vi "Cartesian Product of Lists.vi"(1 "Number of Elements in Each List":i32[](array[numeric])=[2, 2, 3]) -> (0 "Cartesian Product of Lists":i32[][](array[numeric]))   [LabVIEW 2020, in "NI_Gmath.lvlib"]
uses:
  NI_Gmath.lvlib
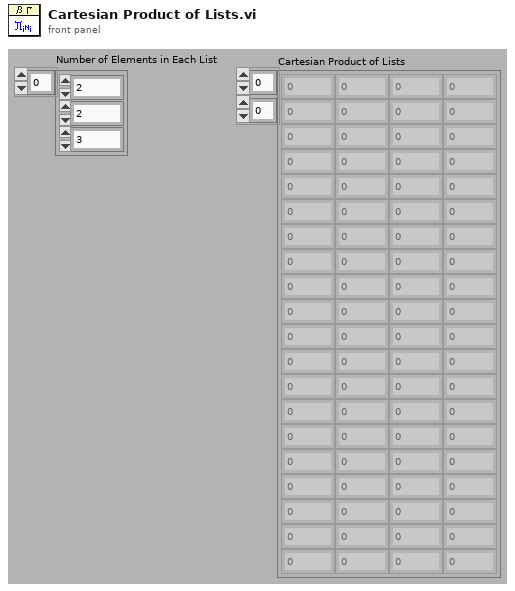
[diagram p1: front panel]
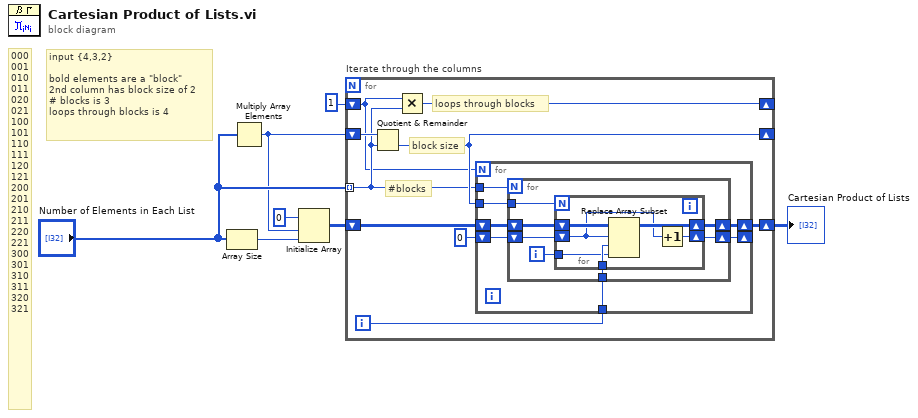
[diagram p0: block diagram]
diagram:
  # "input {4,3,2}\n\nbold elements are a \"block\"\n2nd column has block size of 2\n# blocks is 3\nloops through blocks is 4"
  # "000\n001\n010\n011\n020\n021\n100\n101\n110\n111\n120\n121\n200\n201\n210\n211\n220\n221\n300\n301\n310\n311\n320\n321"
  n1 = Array Size(array="Number of Elements in Each List") -> (size(s)=w3:i32)
  n2 = Multiply Array Elements(1:"Number of Elements in Each List") -> (0:w4:i32)
  n3 = Initialize Array(0, w4, w3) -> (w6:i32[][])
  n4 = for "Iterate through the columns" {
    tunnel: "Number of Elements in Each List" -> [w10] mode=indexing
    shift-right: [w15] -> _
    shift-left: w4 -> [w16]
    shift-right: [w13] -> w1
    shift-left: w6 -> [w14]
    shift-right: [w9] -> _
    shift-left: 1 -> [w8]
    i -> [w12]
    # "loops through blocks"
    # "block size"
    # "#blocks"
    n5 = Quotient & Remainder(x=w16, y=w10) -> (floor(x/y)=w15:i32)  [unwired: 1 out]
    n6 = Multiply(x=w8, y=w10) -> (x*y=w9:i32)
    n7 = for {
      N: w8 -> [_]
      tunnel: w10 -> [w23]
      tunnel: w15 -> [w22]
      shift-right: [w20] -> w13
      shift-left: w14 -> [w21]
      tunnel: w12 -> [w19]
      shift-right: [w17] -> _
      shift-left: 0 -> [w18]
      n8 = for {
        N: w23 -> [_]
        tunnel: w22 -> [w30]
        shift-right: [w28] -> w20
        shift-left: w21 -> [w29]
        tunnel: w19 -> [w27]
        shift-right: [w25] -> w17
        shift-left: w18 -> [w26]
        i -> [w24]
        n9 = for "Fill up a block" {
          N: w30 -> [_]
          shift-right: [w34] -> w28
          shift-left: w29 -> [w36]
          tunnel: w27 -> [w35]
          shift-right: [w32] -> w25
          shift-left: w26 -> [w33]
          tunnel: w24 -> [w31]
          n10 = Replace Array Subset(array=w36, new element=w31, index (row)=w33, index (col)=w35) -> (w34:i32[][])
          n11 = Increment(x=w33) -> (x+1=w32:i32)
        }
      }
    }
  }
  "Cartesian Product of Lists" <- w1
